vi "Embedded Project v2.vi"() -> ()   [LabVIEW 2015]
uses:
  <vilib>/Instr/_visa.llb/Select Event Type.ctl
  <vilib>/Instr/_visa.llb/VISA Configure Serial Port (Instr).vi
panel:
  in  "Tab Control":enum32{"Main", "Misc"}(tab)
  out "Structure\nWarning":bool
  out "Tsunami \nWarning":bool
  out "Earthquake\nWarning":bool
  out "Bridge Stress":dbl[][](graph)
  out "Node 3":bool
  out "Node 2":bool
  out "Node 1":bool
  out "Z Axis":i16[][](graph)
  out "Y Axis":i16[][](graph)
  out "X Axis":i16[][](graph)
  out "Node 1 Water Level":u8(knob) scale=0.0..3.0
  out "Node 2 Water Level":u8(knob) scale=0.0..3.0
  out "Node 3 level":u8(knob) scale=0.0..3.0
  in  "stop":bool
  out "Serial Monitor":string
  in  "COM Port":refnum<visa-resource-name>="COM1"
  out "Output Array":T1(array[cluster])
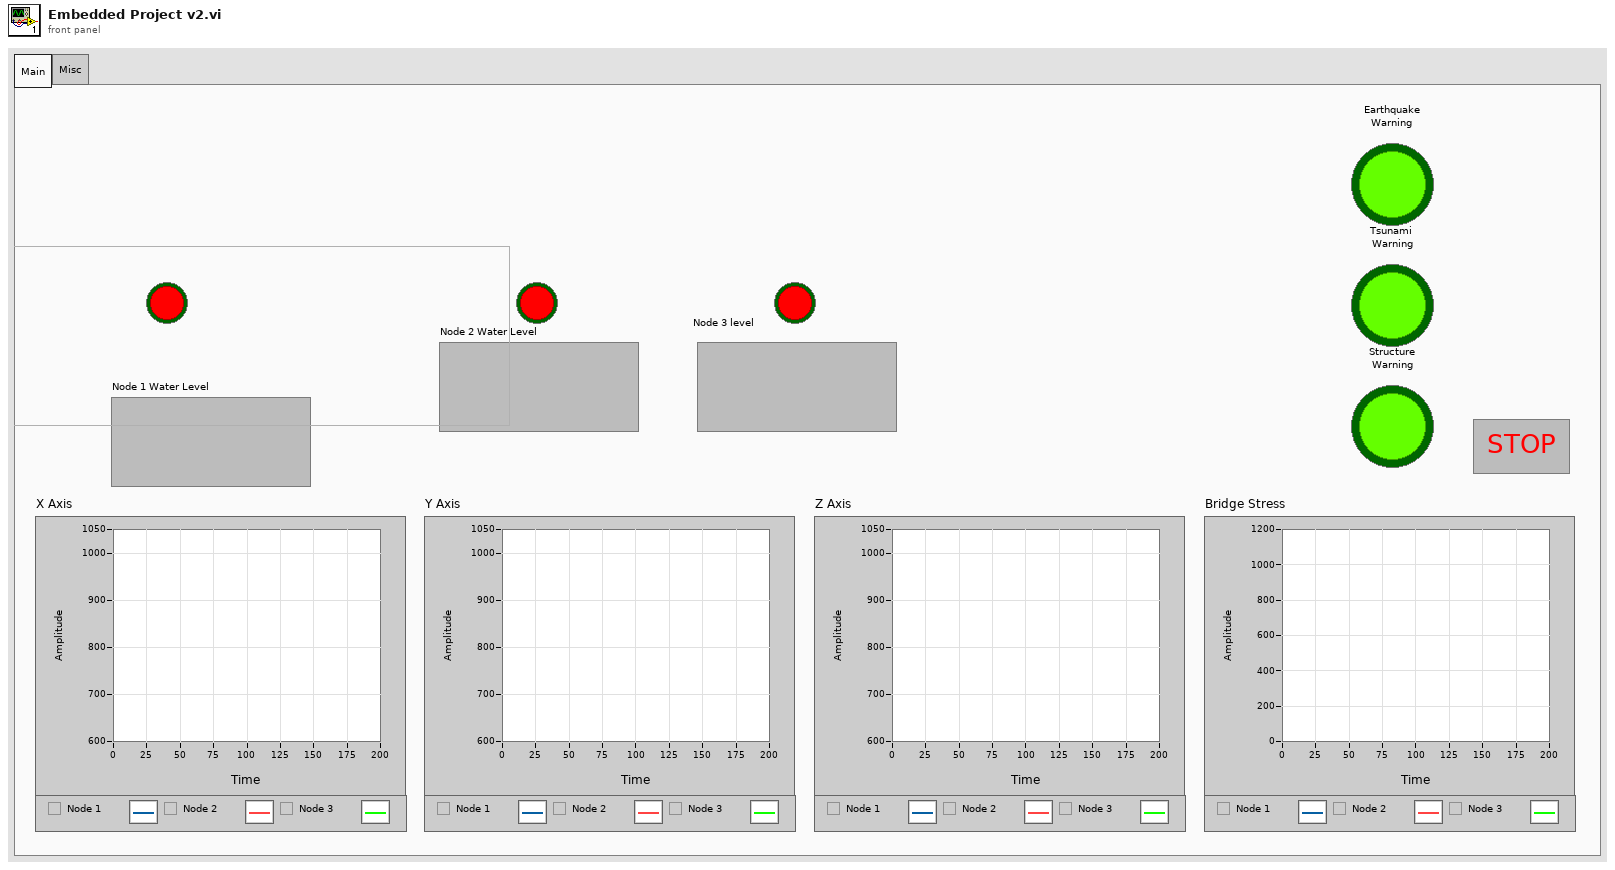
[diagram p1: front panel]
types:
  T1 = cluster{"Node Address":u16, "X Axis":i16, "Y Axis":i16, "Z Axis":i16, "Load Cell":dbl, "Water Level":u8, "Status":bool}[]
  T2 = typedef "Select Event Type.ctl" = u32
  T3 = cluster{"baud rate (9600)":u32, "data bits (8)":u16, "parity (0:none)":enum16{"None", "Odd", "Even", "Mark", "Space"}, "stop bits (10: 1 bit)":u16, "flow control (0:none)":u16}
  T4 = cluster{"Node Address":u16, "X Axis":i16, "Y Axis":i16, "Z Axis":i16, "Load Cell":dbl, "Water Level":u8, "Status":bool}
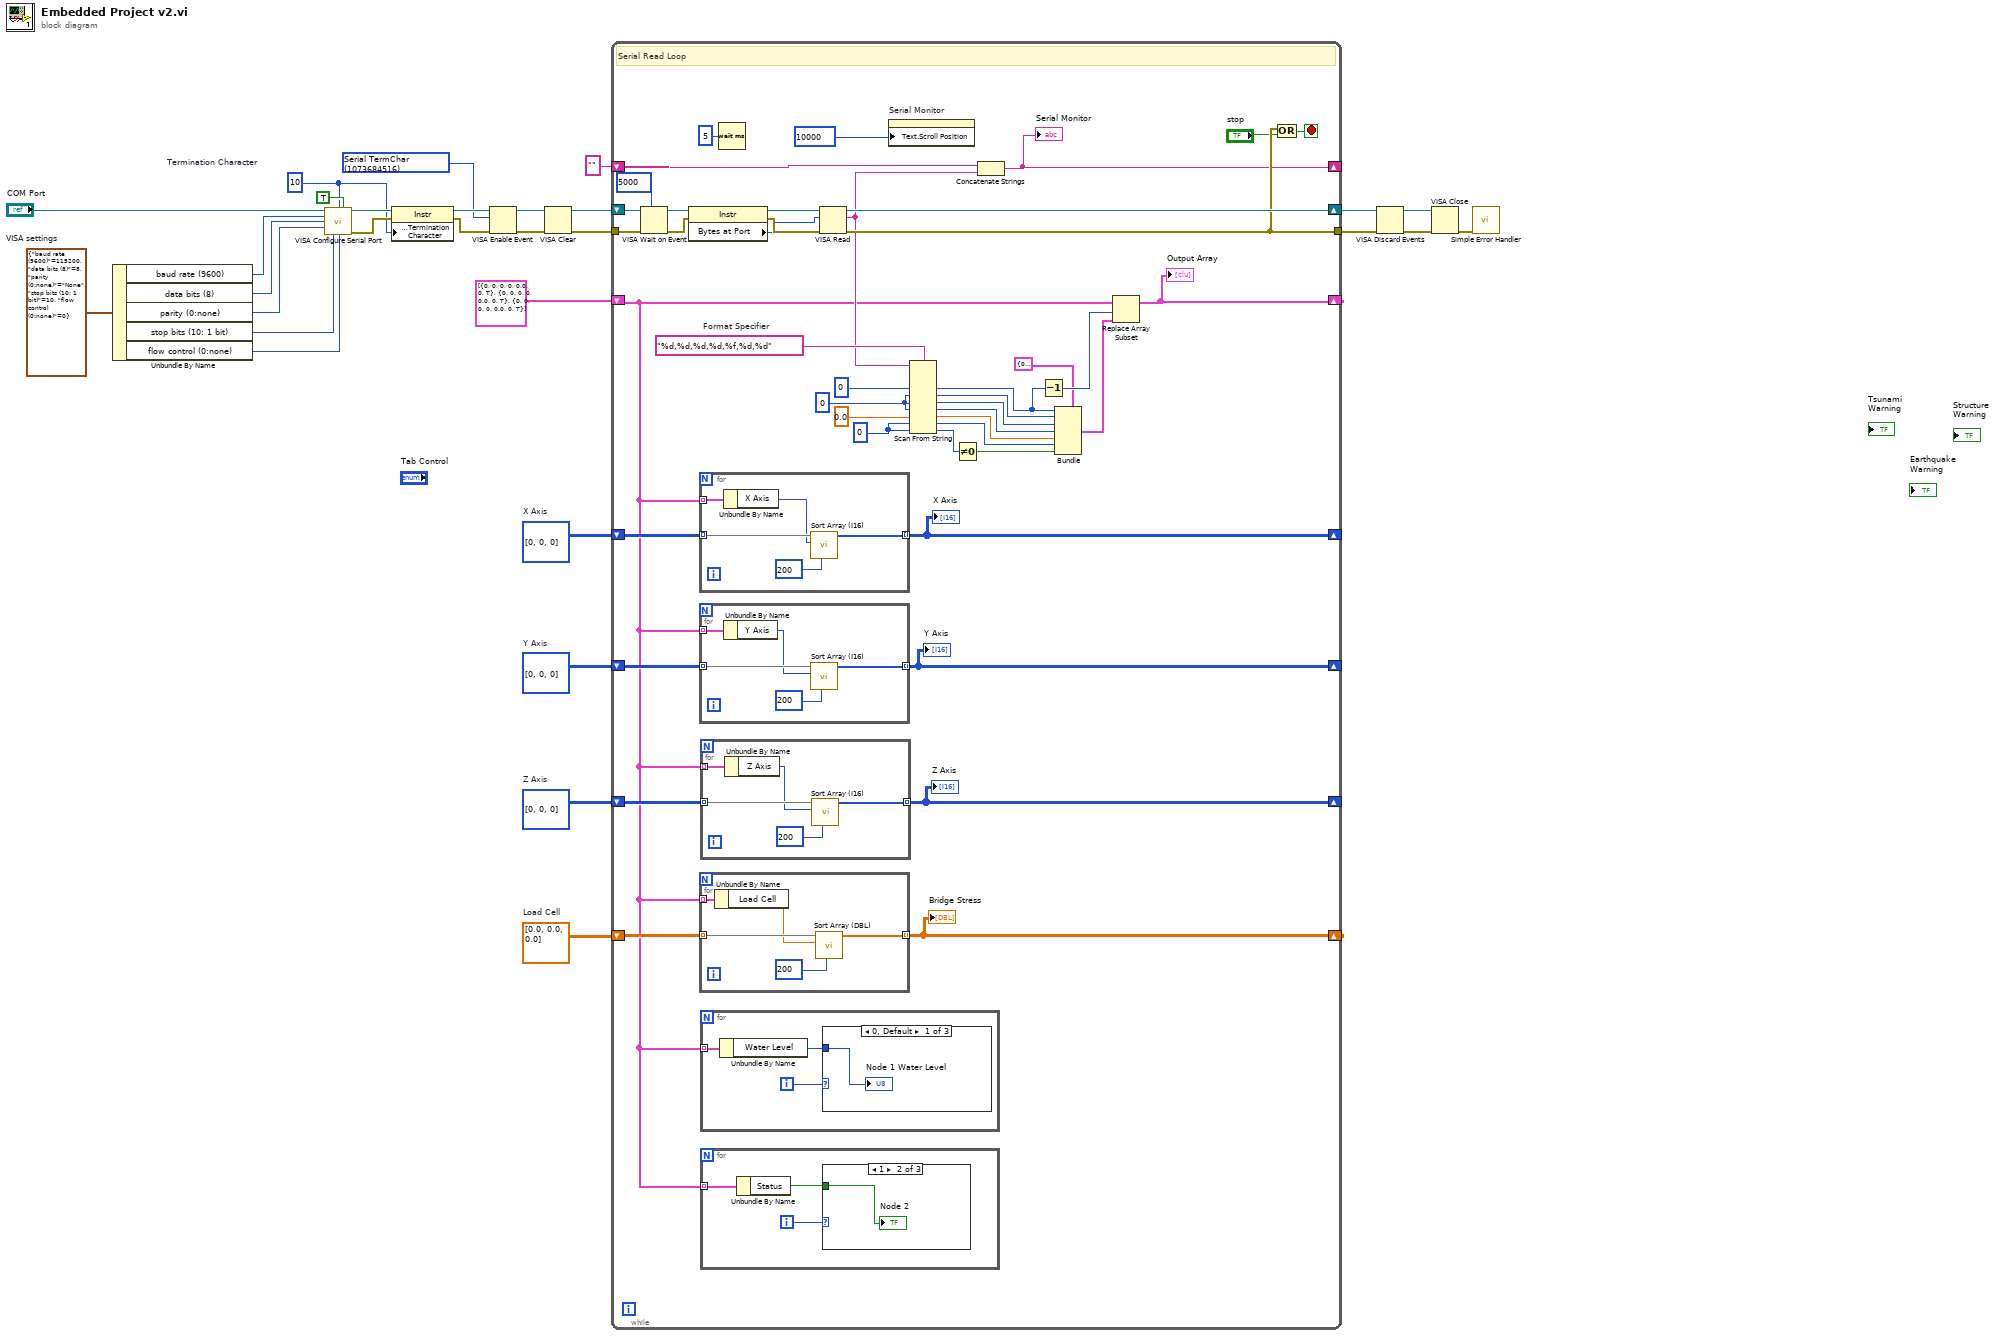
[diagram p0: block diagram]
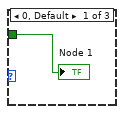
[diagram p2: hidden frame]
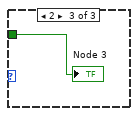
[diagram p3: hidden frame]
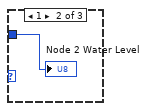
[diagram p4: hidden frame]
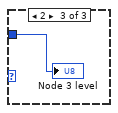
[diagram p5: hidden frame]
diagram:
  w1 = dbl[][] [[0.0], [0.0], [0.0]]  # Load Cell
  w3 = u16[][] [[0], [0], [0]]  # Z Axis
  w4 = u16[][] [[0], [0], [0]]  # Y Axis
  w5 = u16[][] [[0], [0], [0]]  # X Axis
  w15 = T2 1073684516 items=["Service Request"=1073684491, "Trigger"=3221168138, "Clear"=1073684493, "VXI Signal"=1073684512, "VXI/VME Interrupt"=3221168161, "VXI/VME Sysfail"=1073684509, "VXI/VME Sysreset"=1073684510, "GPIB CIC"=1073684498, "GPIB Talk"=1073684499, "GPIB Listen"=1073684500, "PXI Interrupt"=1073684514, "Serial Break"=1073684515, "Serial TermChar"=1073684516, "Serial CTS"=1073684521, "Serial DSR"=1073684522, "Serial DCD"=1073684524, "Serial RI"=1073684526, "Serial Character"=1073684533, "USB Interrupt"=1073684535, "All Enabled"=1073709055] ("Event Type")
  w25 = T3 {"baud rate (9600)"=115200, "data bits (8)"=8, "parity (0:none)"=enum."None", "stop bits (10: 1 bit)"=10, "flow control (0:none)"=0}  # VISA settings
  w18 = u8 10  # Termination Character
  n1 = Unbundle By Name(w25) -> ("baud rate (9600)"=w24:u32, "data bits (8)"=w23:u16, "parity (0:none)"=w22:enum16{"None", "Odd", "Even", "Mark", "Space"}, "stop bits (10: 1 bit)"=w21:u16, "flow control (0:none)"=w20:u16)
  n2 = call-poly "VISA Configure Serial Port"("VISA resource name"="COM Port", "termination char\n(0xA = '\\n' = LF)"=w18, "Enable Termination\nChar (T)"=TRUE ("End Read on Termination Character?"), "baud rate (9600)"=w24, "data bits (8)"=w23, "parity (0:none)"=w22, "stop bits (10: 1 bit)"=w21, "flow control (0:none)"=w20) -> ("VISA resource name out"=w28:refnum<visa-resource-name>, "error out"=w19:errorcluster)  [unwired: 2 in, 4 out]
  n3 = property class="Instr"(reference=w28, error in=w19, "Message Based Settings:Termination Character"=w18) -> (reference out=w16:refnum<visa-resource-name>, error out=w17:errorcluster)
  n4 = VISA Enable Event(8:w17, 10:w15, 11:w16) -> (0:w11:errorcluster, 3:w13:refnum<visa-resource-name>)  [unwired: 1 in]
  n5 = VISA Clear(VISA resource name=w13, error in (no error)=w11) -> (VISA resource name out=w12:refnum<visa-resource-name>, error out=w10:errorcluster)
  n6 = while {
    shift-right: [w72] -> w9
    shift-left: w12 -> [w65]
    tunnel: [w69] -> w6
    shift-right: [w66] -> _
    shift-left: "" -> [w67]
    tunnel: w10 -> [w64]
    shift-right: [w51] -> _
    shift-left: T1 [{"Node Address"=0, "X Axis"=0, "Y Axis"=0, "Z Axis"=0, "Load Cell"=0.0, "Water Level"=0, "Status"=TRUE}, {"Node Address"=0, "X Axis"=0, "Y Axis"=0, "Z Axis"=0, "Load Cell"=0.0, "Water Level"=0, "Status"=TRUE}, {"Node Address"=0, "X Axis"=0, "Y Axis"=0, "Z Axis"=0, "Load Cell"=0.0, "Water Level"=0, "Status"=TRUE}] -> [w30]
    shift-right: [w48] -> _
    shift-left: w5 -> [w49]
    shift-right: [w47] -> _
    shift-left: w4 -> [w46]
    shift-right: [w44] -> _
    shift-left: w3 -> [w45]
    shift-right: [w40] -> _
    shift-left: w1 -> [w42]
    stop <- w70 stop-if-true
    w33 = u8 0 ("default value 6")
    w39 = i16 0 ("default value 1")
    w56 = "%d,%d,%d,%d,%f,%d,%d"  # Format Specifier
    # "Serial Read Loop"
    n7 = VISA Wait on Event(7:u32 5000 ("timeout (0)"), 8:w64, 11:w65) -> (0:w62:errorcluster, 3:w63:refnum<visa-resource-name>)  [unwired: 2 in, 2 out]
    n8 = property class="Instr"(reference=w63, error in=w62) -> (reference out=w61:refnum<visa-resource-name>, error out=w60:errorcluster, "Bytes at Port"=w59:u32)
    n9 = for {
      tunnel: w30 -> [w104] mode=indexing
      tunnel: w49 -> [w103] mode=indexing
      tunnel: [w101] -> w48 mode=indexing
      n10 = Unbundle By Name(w104) -> ("X Axis"=w102:i16)
      n11 = call "Sort Array (I16).vi"("Max Size"=200, "New Element"=w102, "Array In"=w103) -> ("Array Out"=w101:i16[])  [unwired: 8 in]
    }
    "X Axis" <- w48
    n12 = for {
      tunnel: w46 -> [w99] mode=indexing
      tunnel: [w98] -> w47 mode=indexing
      tunnel: w30 -> [w95] mode=indexing
      n13 = Unbundle By Name(w95) -> ("Y Axis"=w96:i16)
      n14 = call "Sort Array (I16).vi"("Max Size"=200, "New Element"=w96, "Array In"=w99) -> ("Array Out"=w98:i16[])  [unwired: 8 in]
    }
    "Y Axis" <- w47
    n15 = for {
      tunnel: [w88] -> w40 mode=indexing
      tunnel: w42 -> [w87] mode=indexing
      tunnel: w30 -> [w89] mode=indexing
      n16 = Unbundle By Name(w89) -> ("Load Cell"=w86:dbl)
      n17 = call "Sort Array (DBL).vi"("Max Size"=200, "New Element"=w86, "Array In"=w87) -> ("Array Out"=w88:dbl[])  [unwired: 8 in]
    }
    "Bridge Stress" <- w40
    n18 = for {
      tunnel: [w94] -> w44 mode=indexing
      tunnel: w45 -> [w92] mode=indexing
      tunnel: w30 -> [w90] mode=indexing
      n19 = Unbundle By Name(w90) -> ("Z Axis"=w91:i16)
      n20 = call "Sort Array (I16).vi"("Max Size"=200, "New Element"=w91, "Array In"=w92) -> ("Array Out"=w94:i16[])  [unwired: 8 in]
    }
    "Z Axis" <- w44
    n21 = for {
      tunnel: w30 -> [w81] mode=indexing
      i -> [w80]
      n22 = Unbundle By Name(w81) -> ("Water Level"=w79:u8)
      n23 = case shown="0, Default" w80 {
        tunnel: w79 -> [w82 w83 w84]
        frame 0, Default {
          "Node 1 Water Level" <- w82
        }
        frame 1 {
          "Node 2 Water Level" <- w83
        }
        frame 2 {
          "Node 3 level" <- w84
        }
      }
    }
    n24 = for {
      tunnel: w30 -> [w75] mode=indexing
      i -> [w74]
      n25 = Unbundle By Name(w75) -> ("Status"=w73:bool)
      n26 = case shown="1" w74 {
        tunnel: w73 -> [w76 w77 w78]
        frame 0, Default {
          "Node 1" <- w76
        }
        frame 1 {
          "Node 2" <- w77
        }
        frame 2 {
          "Node 3" <- w78
        }
      }
    }
    n27 = Wait (ms)(milliseconds to wait=u32 5) -> ()  [unwired: 1 out]
    n28 = VISA Read(VISA resource name=w61, byte count=w59, error in (no error)=w60) -> (VISA resource name out=w72:refnum<visa-resource-name>, read buffer=w54:string, error out=w69:errorcluster)  [unwired: 1 out]
    n29 = property on="Serial Monitor" class="Str"("Text.Scroll Position"=u32 10000) -> ()  [unwired: 2 in, 2 out]
    n30 = Scan From String(format string=w56, input string=w54, default 1=u16 0 ("default value 1"), default 2=w39, default 3=w39, default 4=w39, default 5=0.0 ("default value 1"), default 6=w33, default 7=w33) -> (output 1=w53:u16, output 2=w57:i16, output 3=w37:i16, output 4=w36:i16, output 5=w35:dbl, output 6=w34:u8, output 7=w32:u8)  [unwired: 2 in, 3 out]
    n31 = Not Equal To 0?(x=w32) -> (x != 0?=w31:bool)
    n32 = Concatenate Strings(w67, w54) -> (w66:string)
    "Serial Monitor" <- w66
    n33 = Decrement(x=w53) -> (x-1=w52:u16)
    n34 = Bundle(cluster=T4 {"Node Address"=0, "X Axis"=0, "Y Axis"=0, "Z Axis"=0, "Load Cell"=0.0, "Water Level"=0, "Status"=TRUE} ("Node 4"), "Node Address"=w53, "X Axis"=w57, "Y Axis"=w37, "Z Axis"=w36, "Load Cell"=w35, "Water Level"=w34, "Status"=w31) -> (w50:T4)
    n35 = Replace Array Subset(array=w30, new element=w50, index=w52) -> (w51:T1)
    "Output Array" <- w51
    n36 = Or(x=w69, y="stop") -> (x .or. y?=w70:bool)
  }
  n37 = VISA Discard Events(8:w6, 11:w9) -> (0:w7:errorcluster, 3:w8:refnum<visa-resource-name>)  [unwired: 2 in]
  n38 = VISA Close(VISA resource name=w8, error in (no error)=w7) -> (error out=w26:errorcluster)
  n39 = call <vilib>:"Simple Error Handler.vi"("error in (no error)"=w26) -> ()  [unwired: 1 in, 8 out]
